vi "Test TCPConnection Process Kill.vi"   [LabVIEW 2013]
uses:
  source/Server/Connection/TCPConnection.lvclass
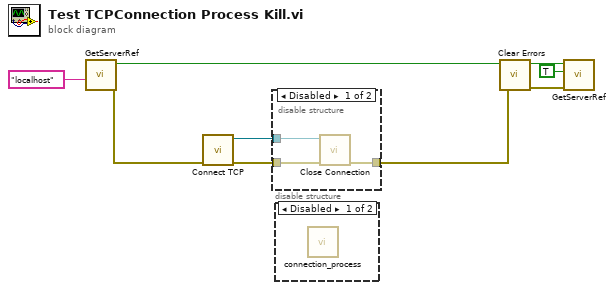
[diagram p0: block diagram]
diagram:
  n1 = call "GetServerRef.vi"("address (localhost)"="localhost") -> ("error out"=w3:errorcluster, "Created"=w6:bool)  [unwired: 7 in, 2 out]
  n2 = call "Connect TCP.vi"("error in (no error)"=w3) -> ("error out"=w7:errorcluster, "TCPConnection out"=w8:refnum<class "TCPConnection.lvclass">)  [unwired: 9 in]
  n3 = disable-structure shown="Disabled" {
    disable-tunnel: w8 -> [w11 _]
    disable-tunnel: w7 -> [w10 w12]
    disable-tunnel: [w9 w12] -> w2
    frame Disabled {
      n4 = call-dynamic "Close Connection.vi"("error in (no error)"=w10, "TCPConnection in"=w11) -> ("error out"=w9:errorcluster)  [unwired: 8 in, 1 out]
    }
    frame Enabled {
    }
  }
  n5 = disable-structure shown="Disabled" {
    frame Disabled {
      n6 = call "connection_process.vi"() -> ()  [unwired: 12 in]
    }
    frame Enabled {
    }
  }
  n7 = call <vilib>:"Clear Errors.vi"("error in (no error)"=w2) -> ("error out"=w1:errorcluster)  [unwired: 6 in]
  n8 = call "GetServerRef.vi"("error in"=w1, "Force Destroy (F)"=TRUE, "Destroy (F)"=w6) -> ()  [unwired: 5 in, 4 out]
